vi "PH_BL-Master.set Boolean Status Service Subscriber.vi"(0 "i ref in":refnum<vi>, 1 "Ref Switch and 6P State Instances":refnum<vi>, 2 "Force Sensor Instances":refnum<vi>, 5 "error in":errorcluster, 6 "Ref Switch GUI Instances":refnum<vi>, 7 "Boolean Status Service Subscriber GUI Refs":refnum<vi>[](array[refnum]), 8 "Ref 6P Switch Instances":refnum<vi>, 10 "Ref BB Instances":refnum<vi>, 12 "Ref Switch Instances":refnum<vi>) -> (14 "i ref out":refnum<vi>, 19 "error out":errorcluster)   [LabVIEW 2014, in "PH_BL-Master.lvlib"]
uses:
  PH_BL-Master.lvlib
  PH_Basics/PH_StatusHandler/PH_StatusHandler.Status.ctl
  PH_BL-Master.Status Subscriber Class.ctl
  PH_Basics/PH_StatusHandler/PH_StatusHandler.lvlib
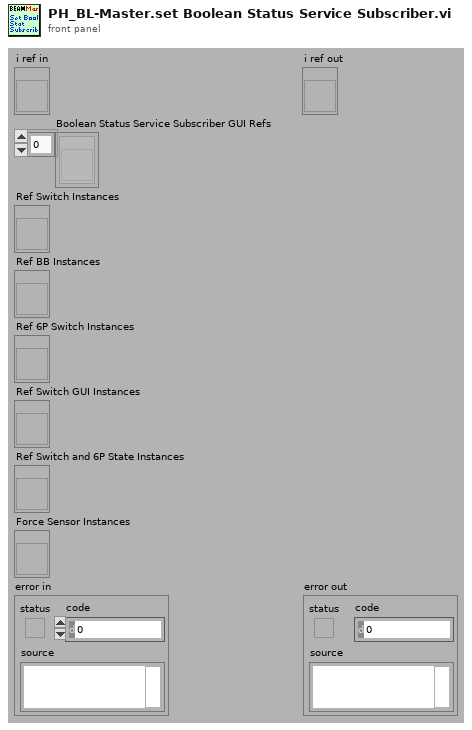
[diagram p1: front panel]
types:
  T1 = typedef "PH_StatusHandler.lvlib/PH_StatusHandler.Status.ctl" = i16
  T2 = typedef "PH_BL-Master.lvlib/PH_BL-Master.Status Subscriber Class.ctl" = enum16{"unknown", "Switch", "BB", "6P Switch", "Switch GUI", "Switch and 6P State", "Force Sensor"}
  T3 = cluster{"GUI Ref":refnum<vi>, "Status":T1, "no Link?":bool, "Status Subscriber Class":T2}
  T4 = typedef "PH_BL-Master.lvlib/PH_BL-Master.i attribute.ctl" = cluster{"Remote controlled":bool, "Boolean Condition Service Subscriber":refnum<vi>[], "Picture Condition Service Subscriber":refnum<vi>[], "R2S":cluster{"GUI Ref":refnum<vi>, "State":bool}, "Vacua":cluster{"GUI Ref":refnum<vi>, "Limit":dbl, "Curr Value":dbl, "in range":bool}[], "O2 Inspection":cluster{"GUI Ref":refnum<vi>, "Concentration":dbl, "State":T1}[], "Boolean Status Service Subscriber":cluster{"GUI Ref":refnum<vi>, "Status":T1, "no Link?":bool, "Status Subscriber Class":T2}[], "Picture Status Service Subscriber":cluster{"GUI Ref":refnum<vi>, "Status":T1, "no Link?":bool, "Status Subscriber Class":T2}[], "6P 4Q Service Subscriber":cluster{"GUI Ref":refnum<vi>, "Selector":T5, "no Link?":bool}[], "Index of latest 6P 4Q changing Instance":i32, "Index of latest Picture Status changing Instance":i32, "Index of latest Boolean Status changing Instance":i32, "Vision ID on same Node":string, "Start Phase over?":bool, "GUI Ref Delete":refnum<vi>}
  T5 = typedef "PH_4_Pos_Selector.lvlib/PH_4_Pos_Selector.Position Selector.ctl" = u16
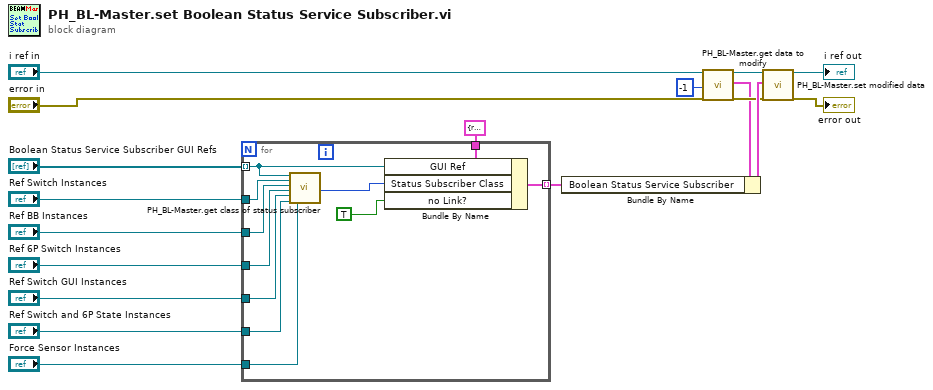
[diagram p0: block diagram]
diagram:
  n1 = for {
    tunnel: [w29] -> w7 mode=indexing
    tunnel: "Boolean Status Service Subscriber GUI Refs" -> [w26] mode=indexing
    tunnel: T3 {"GUI Ref"=refnum, "Status"=0, "no Link?"=FALSE, "Status Subscriber Class"=enum."unknown"} ("Bool Stat Serv Dummy") -> [w28]
    tunnel: "Ref Switch Instances" -> [w25]
    tunnel: "Ref BB Instances" -> [w24]
    tunnel: "Ref 6P Switch Instances" -> [w23]
    tunnel: "Ref Switch and 6P State Instances" -> [w22]
    tunnel: "Ref Switch GUI Instances" -> [w21]
    tunnel: "Force Sensor Instances" -> [w19]
    n2 = call "PH_BL-Master.get class of status subscriber.vi"("GUI Ref"=w26, "Ref Switch Instances"=w25, "Ref BB Instances"=w24, "Ref 6P Switch Instances"=w23, "Ref Switch GUI Instances"=w21, "Ref Switch and 6P State Instances"=w22, "Force Sensor Instances"=w19) -> ("Status Subscriber Class"=w27:T2)  [unwired: 12 in]
    n3 = Bundle By Name(cluster=w28, "GUI Ref"=w26, "Status Subscriber Class"=w27, "no Link?"=TRUE) -> (w29:T3)
  }
  n4 = call "PH_BL-Master.get data to modify.vi"("i ref in"="i ref in", "ms timeout (10000)"=-1, "error in (no error)"="error in") -> ("i ref out"=w15:refnum<vi>, "i attribute"=w10:T4, "error out"=w13:errorcluster)  [unwired: 13 in, 1 out]
  n5 = Bundle By Name(cluster=w10, "Boolean Status Service Subscriber"=w7) -> (w16:T4)
  n6 = call "PH_BL-Master.set modified data.vi"("i ref in"=w15, "i attribute"=w16, "error in (no error)"=w13) -> ("i ref out"=→"i ref out":refnum<vi>, "error out"=→"error out":errorcluster)  [unwired: 15 in]
